vi "Write.vi"(10 "Boolean Array":bool[](array[boolean]), 11 "Boolean Array in":refnum<class "Boolean Array.lvclass">) -> (3 "Boolean Array out":refnum<class "Boolean Array.lvclass">)   [LabVIEW 2020, in "Data.lvlib" / "Boolean Array.lvclass"]
doc: "Write Boolean Array."
uses:
  Boolean Array.lvclass
  Boolean Array.lvclass/Boolean Array.ctl
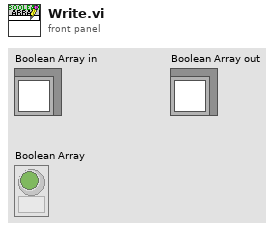
[diagram p1: front panel]
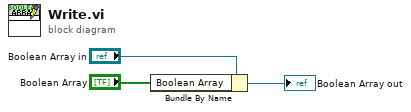
[diagram p0: block diagram]
diagram:
  n1 = Bundle By Name(cluster="Boolean Array in", "Boolean Array"="Boolean Array") -> (→"Boolean Array out":refnum<class "Boolean Array.lvclass">)
